vi "Module Cleanup.vi"(8 "error in (no error)":errorcluster, 11 "ToggleTestModule in":refnum<class "ToggleTestModule.lvclass">) -> (0 "error out":errorcluster, 3 "ToggleTestModule out":refnum<class "ToggleTestModule.lvclass">)   [LabVIEW 2020, in "VolatusScratch.lvlib" / "ToggleTestModule.lvclass"]
uses:
  ToggleTestModule.lvclass
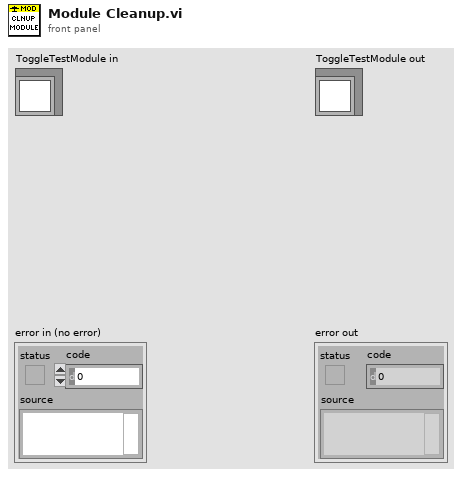
[diagram p1: front panel]
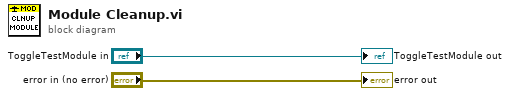
[diagram p0: block diagram]
diagram:
  "error out" <- "error in (no error)"
  "ToggleTestModule out" <- "ToggleTestModule in"
